vi "call.vi"(7 "LabVIEW Web Service Request":refnum<class "Web Request.lvclass">) -> ()   [LabVIEW 2015]
uses:
  <vilib>/wsapi/Web Request.lvclass
  Source/Classes/Server/Send Request (Async).vi
  Source/Classes/Server/Send Request (Sync).vi
  Source/Classes/Server/JSONRPC Server.lvclass
panel:
  # "Use the Web Service Request input terminal to call the VIs on the Web Services palette. Do not remove it from the connector pane unless you don't need access to the palette."
  # "Each additional control wired to the connector pane will be available as an input in the URL. To include an indicator in terminal-mode output (the default setting), it must also be wired to the connector pane."
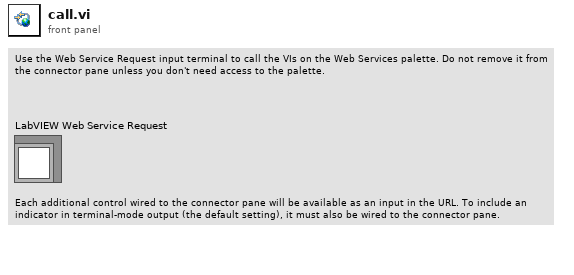
[diagram p1: front panel]
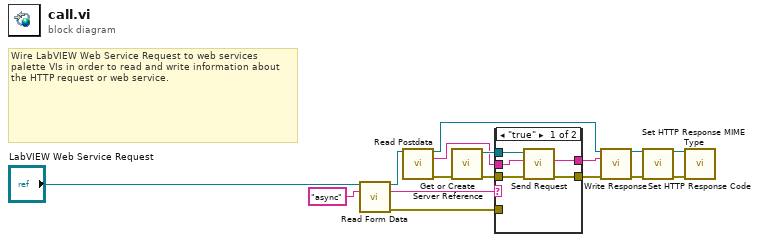
[diagram p0: block diagram]
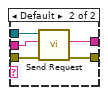
[diagram p2: hidden frame]
diagram:
  # "Wire LabVIEW Web Service Request to web services palette VIs in order to read and write information about the HTTP request or web service."
  n1 = call <vilib>:"Read Form Data.vi"("LabVIEW Web Service Request"="LabVIEW Web Service Request", "key"="async") -> ("LabVIEW Web Service Request out"=w7:refnum<class "Web Request.lvclass">, "value"=w10:string, "error out"=w9:errorcluster)  [unwired: 10 in, 1 out]
  n2 = call <vilib>:"Read Postdata.vi"("LabVIEW Web Service Request"=w7) -> ("LabVIEW Web Service Request out"=w1:refnum<class "Web Request.lvclass">, "postdata"=w15:string, "error out"=w6:errorcluster)  [unwired: 12 in]
  n3 = call "Get or Create Server Reference.vi"("error in (no error)"=w6) -> ("error out"=w5:errorcluster, "Server Out"=w16:refnum<class "JSONRPC Server.lvclass">)  [unwired: 9 in]
  n4 = case shown="\"true\"" w10 {
    tunnel: w16 -> [w21 w26]
    tunnel: w15 -> [w20 w25]
    tunnel: [w19 w24] -> w14
    tunnel: w9 -> [_ _]
    tunnel: w5 -> [w18 w23]
    tunnel: [w17 w22] -> w4
    frame "true" {
      n5 = call-poly "Send Request.vi"("error in (no error)"=w18, "JSON Request String"=w20, "Server in"=w21) -> ("error out"=w17:errorcluster, "id value"=w19:string)  [unwired: 5 in, 2 out]
    }
    frame Default {
      n6 = call-poly "Send Request.vi"("error in (no error)"=w23, "JSON Request String"=w25, "JSONRPC Server in"=w26) -> ("error out"=w22:errorcluster, "JSON Response String"=w24:string)  [unwired: 6 in, 1 out]
    }
  }
  n7 = call <vilib>:"Write Response.vi"("LabVIEW Web Service Request"=w1, "response string"=w14, "error in (no error)"=w4) -> ("LabVIEW Web Service Request out"=w2:refnum<class "Web Request.lvclass">, "error out"=w3:errorcluster)  [unwired: 11 in]
  n8 = call <vilib>:"Set HTTP Response MIME Type.vi"("LabVIEW Web Service Request"=w2, "error in (no error)"=w3) -> ("LabVIEW Web Service Request out"=w13:refnum<class "Web Request.lvclass">, "error out"=w12:errorcluster)  [unwired: 12 in]
  n9 = call <vilib>:"Set HTTP Response Code.vi"("LabVIEW Web Service Request"=w13, "error in (no error)"=w12) -> ()  [unwired: 12 in, 2 out]
